vi "DROPBEAR_Model_Updating_Main.vi"() -> ()   [LabVIEW 2021, in "DROPBEAR_Model_Updating.lvclass"]
uses:
  DROPBEAR_Model_Updating.lvclass
panel:
  in  "Stop":bool
  out "Cycle time":dbl
  out "Freqeuncy":dynamicdata(graph)
  out "Nodal":dynamicdata(graph)
  out "Meter":dynamicdata(graph)
  in  "Program Controls":T1={"Frequency KF"=TRUE, "Pinned State KF"=TRUE, "FFT Bounding"=TRUE, "Filter Constants Frequency"={"Measurement Variance"=0.4, "State Variance"=0.01, "Threshold"=1000000000.0}, "Filter Constants Position"={"Measurement Variance"=0.09, "State Variance"=0.01, "Threshold"=0.019999999999999997}, "Moving Window Size"=10.0} {"Filter Constants Frequency"."Measurement Variance" min=0.0 step=0.001}
  in  "Simulation Parameters input controls":T2={"Eigensolver "=enum."LEMP", "Models Forcasted"=3, "Max Roller Velocity"=3.32, "Max Roller Position Percent"=0.43, "Min Roller Position Percent"=0.155}
  in  "Mockbear input controls":T3={"Dataset"="test7", "Resample Method"=enum."Auto Resample"}
  in  "Modeling Parameters input controls":T4={"beam_length"=0.3525, "youngs_modulus"=209500000000.0, "torsion_spring"=0.0, "beam_height"=0.00635, "beam_width"=0.0508, "beam_density"=7900.0, "number_of_FEA_nodes"=40, "accelerometer_mass"=0.055}
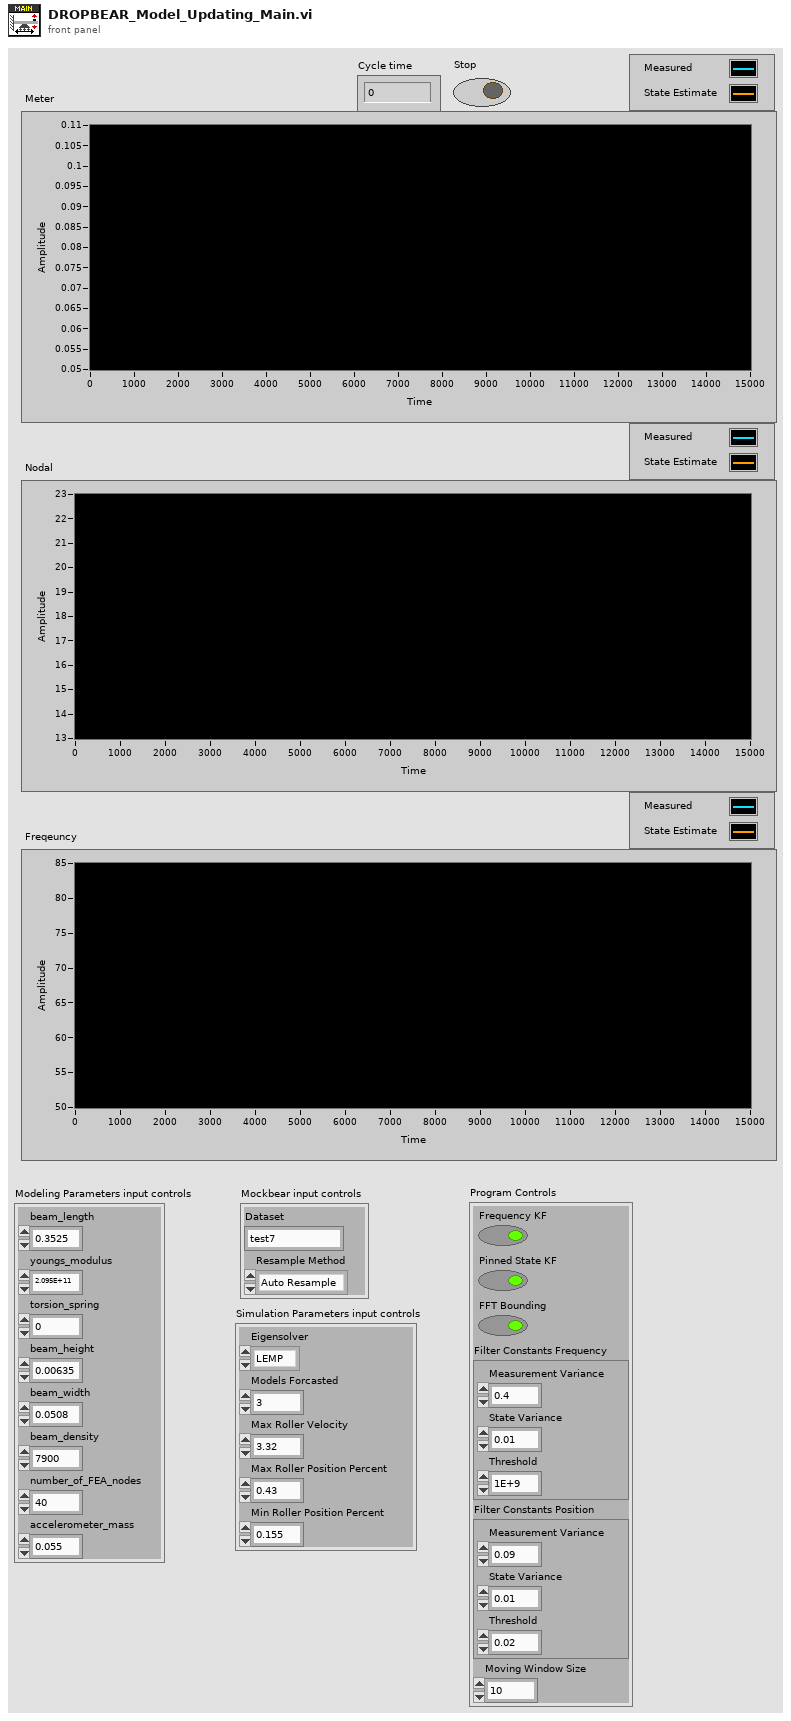
[diagram p1: front panel]
types:
  T1 = cluster{"Frequency KF":bool, "Pinned State KF":bool, "FFT Bounding":bool, "Filter Constants Frequency":cluster{"Measurement Variance":dbl, "State Variance":dbl, "Threshold":dbl}, "Filter Constants Position":cluster{"Measurement Variance":dbl, "State Variance":dbl, "Threshold":dbl}, "Moving Window Size":dbl}
  T2 = cluster{"Eigensolver ":enum16{"LabVIEW Cholesky", "LabVIEW General", "LabVIEW Inverse", "LEMP"}, "Models Forcasted":i32, "Max Roller Velocity":dbl, "Max Roller Position Percent":dbl, "Min Roller Position Percent":dbl}
  T3 = cluster{"Dataset":string, "Resample Method":enum16{"Recorded", "Auto Resample", "Custom Resample"}}
  T4 = cluster{"beam_length":dbl, "youngs_modulus":dbl, "torsion_spring":dbl, "beam_height":dbl, "beam_width":dbl, "beam_density":dbl, "number_of_FEA_nodes":i32, "accelerometer_mass":dbl}
  T5 = cluster{"Modeling Parameters input controls":cluster{"beam_length":dbl, "youngs_modulus":dbl, "torsion_spring":dbl, "beam_height":dbl, "beam_width":dbl, "beam_density":dbl, "number_of_FEA_nodes":i32, "accelerometer_mass":dbl}, "Mockbear input controls":cluster{"Dataset":string, "Resample Method":enum16{"Recorded", "Auto Resample", "Custom Resample"}}, "Simulation Parameters input controls":cluster{"Eigensolver ":enum16{"LabVIEW Cholesky", "LabVIEW General", "LabVIEW Inverse", "LEMP"}, "Models Forcasted":i32, "Max Roller Velocity":dbl, "Max Roller Position Percent":dbl, "Min Roller Position Percent":dbl}, "Program Controls":cluster{"Frequency KF":bool, "Pinned State KF":bool, "FFT Bounding":bool, "Filter Constants Frequency":cluster{"Measurement Variance":dbl, "State Variance":dbl, "Threshold":dbl}, "Filter Constants Position":cluster{"Measurement Variance":dbl, "State Variance":dbl, "Threshold":dbl}, "Moving Window Size":dbl}}
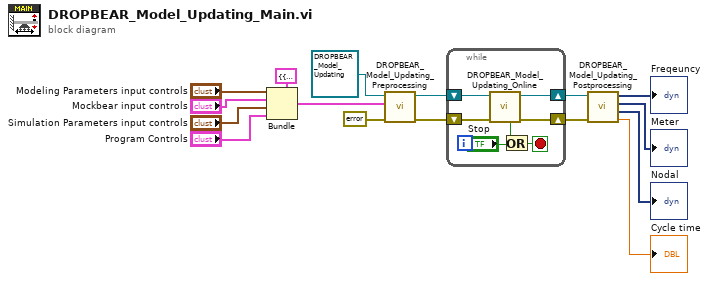
[diagram p0: block diagram]
diagram:
  n1 = Bundle(cluster=T5 {"Modeling Parameters input controls"={"beam_length"=0.0, "youngs_modulus"=0.0, "torsion_spring"=0.0, "beam_height"=0.0, "beam_width"=0.0, "beam_density"=0.0, "number_of_FEA_nodes"=0, "accelerometer_mass"=0.0}, "Mockbear input controls"={"Dataset"="", "Resample Method"=enum."Recorded"}, "Simulation Parameters input controls"={"Eigensolver "=enum."LEMP", "Models Forcasted"=0, "Max Roller Velocity"=0.0, "Max Roller Position Percent"=0.43, "Min Roller Position Percent"=0.155}, "Program Controls"={"Frequency KF"=TRUE, "Pinned State KF"=TRUE, "FFT Bounding"=TRUE, "Filter Constants Frequency"={"Measurement Variance"=0.0, "State Variance"=0.0, "Threshold"=0.0}, "Filter Constants Position"={"Measurement Variance"=0.0, "State Variance"=0.0, "Threshold"=0.0}, "Moving Window Size"=0.0}} ("Setup Parameters and Controls"), "Modeling Parameters input controls"="Modeling Parameters input controls", "Mockbear input controls"="Mockbear input controls", "Simulation Parameters input controls"="Simulation Parameters input controls", "Program Controls"="Program Controls") -> (w10:T5)
  n2 = call-dynamic "DROPBEAR_Model_Updating_Preprocessing.vi"("error in (no error)"=errorcluster {"status"=FALSE, "code"=0, "source"=""}, "Setup Parameters and Controls"=w10, "DROPBEAR_Model_Updating in"=refnum<class "DROPBEAR_Model_Updating.lvclass"> refnum ("DROPBEAR_Model_Updating.lvclass")) -> ("error out"=w8:errorcluster, "DROPBEAR_Model_Updating out"=w7:refnum<class "DROPBEAR_Model_Updating.lvclass">)  [unwired: 7 in]
  n3 = while {
    shift-right: [w21] -> w6
    shift-left: w7 -> [w23]
    shift-right: [w20] -> w1
    shift-left: w8 -> [w22]
    stop <- w19 stop-if-true
    n4 = call-dynamic "DROPBEAR_Model_Updating_Online.vi"("error in (no error)"=w22, "DROPBEAR_Model_Updating in"=w23) -> ("error out"=w20:errorcluster, "DROPBEAR_Model_Updating out"=w21:refnum<class "DROPBEAR_Model_Updating.lvclass">, "looping"=w18:bool)  [unwired: 7 in]
    n5 = Or(x=w18, y="Stop") -> (x .or. y?=w19:bool)
  }
  n6 = call-dynamic "DROPBEAR_Model_Updating_Postprocessing.vi"("error in (no error)"=w1, "DROPBEAR_Model_Updating in"=w6) -> ("Cycle time"=→"Cycle time":dbl, "Nodal"=→"Nodal":dynamicdata, "Meter"=→"Meter":dynamicdata, "Frequency"=→"Freqeuncy":dynamicdata)  [unwired: 6 in]
